vi "ASK_judgement.vi"(8 "error in (no error)":errorcluster caption="错误输入（无错误）", 10 "input_data":dbl[](array[numeric]) format="%#_13g", 11 "PathIn":path) -> (0 "error out":errorcluster caption="错误输出", 2 "judge_data":dbl[](array[numeric]), 3 "PathOut":path)   [LabVIEW 2015]
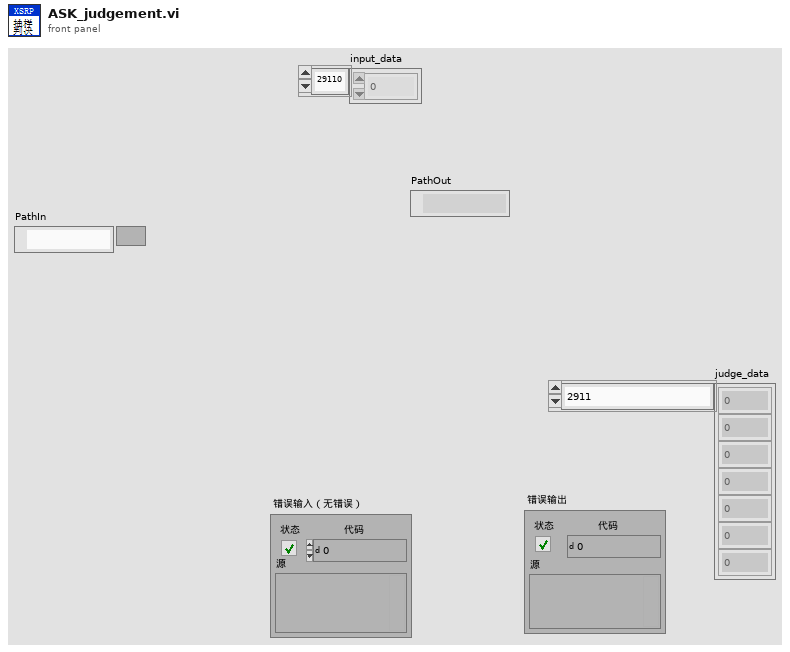
[diagram p1: front panel]
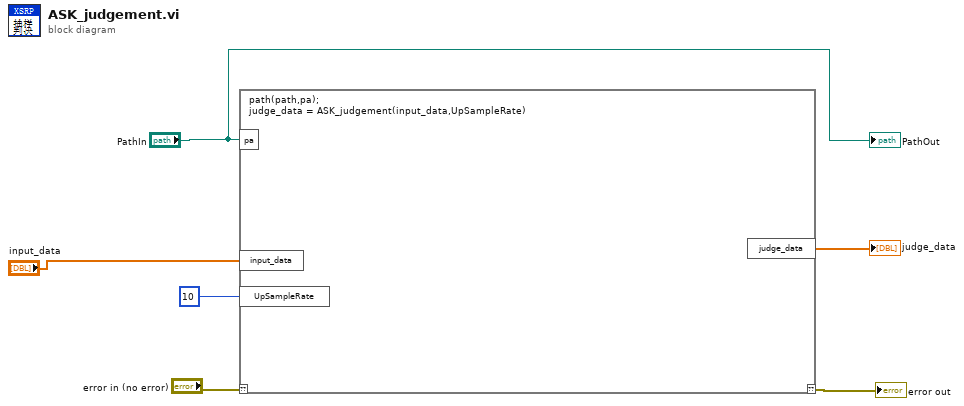
[diagram p0: block diagram]
diagram:
  n1 = script code="path(path,pa);\njudge_data = ASK_judgement(input_data,UpSampleRate)"("??"="error in (no error)", "pa"="PathIn", "input_data"="input_data", "UpSampleRate"=10) -> ("??"=→"error out":errorcluster, "judge_data"=→"judge_data":dbl[])
  "PathOut" <- "PathIn"
